vi "LINX - Blink - TCP Interface.vi"() -> ()   [LabVIEW 2011, in "LVH-LINX.lvlib"]
doc: "Blink and LED attached to a digital output channel of a LINX device."
uses:
  vi.lib/LabVIEW Hacker/LINX/LVH-LINX.lvlib
  vi.lib/LabVIEW Hacker/LINX/Private/Device/Type Defs/TCP Config.ctl
  vi.lib/LabVIEW Hacker/LINX/Private/Type Defs/Interface.ctl
  vi.lib/LabVIEW Hacker/LINX/Private/Device/Device.lvlib
panel:
  in  "TCP Configuration":T1
  out "LED Value":bool
  in  "Digital Output Channel":u8=13
  out "Loop Rate (Hz)":u32
  in  "Stop Button":bool
  # "LINX Device Settings"
  # "LED Value"
  # "Circuit Schematic"
  # "Blink (TCP Interface)\n\nThis example demonstrates how to blink an LED on a LINX device connected to \nthe host computer using TCP.\n\nInstructions\n1. Select the IP Address  and Port associated with the LINX Device.\n2. Select the Digital Pin connected to the LED.\n3. Click the Run Arrow."
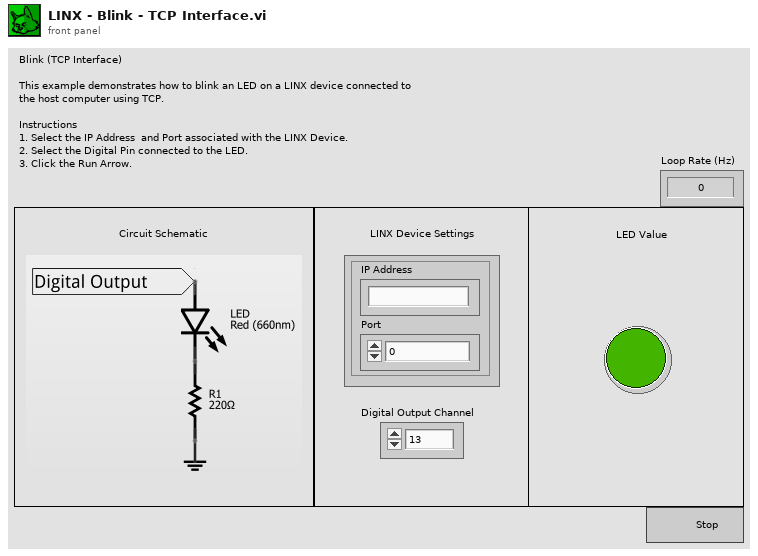
[diagram p1: front panel]
types:
  T1 = typedef "LVH-LINX.lvlib/Device.lvlib/TCP Config.ctl" = cluster{"IP Address":string, "Port":u16}
  T2 = typedef "LVH-LINX.lvlib/Interface.ctl" = enum16{"Serial", "TCP"}
  T3 = typedef "LVH-LINX.lvlib/LINX Ref.ctl" = cluster{"Platform":T4, "Interface":T2, "LINX Device Config":T5}
  T4 = typedef "LVH-LINX.lvlib/Platform.ctl" = enum16{"LINX", "myRIO"}
  T5 = typedef "LVH-LINX.lvlib/Device.lvlib/LINX Device Config.ctl" = cluster{"Interface":T2, "COM Port":refnum<visa-resource-name>, "TCP Configuration":T1, "Device Family":T6, "Device ID":u8, "Device Name":string, "TCP Ref":refnum<k5>}
  T6 = typedef "LVH-LINX.lvlib/Device Family.ctl" = enum8{"National Instruments", "Digilent", "Arduino"}
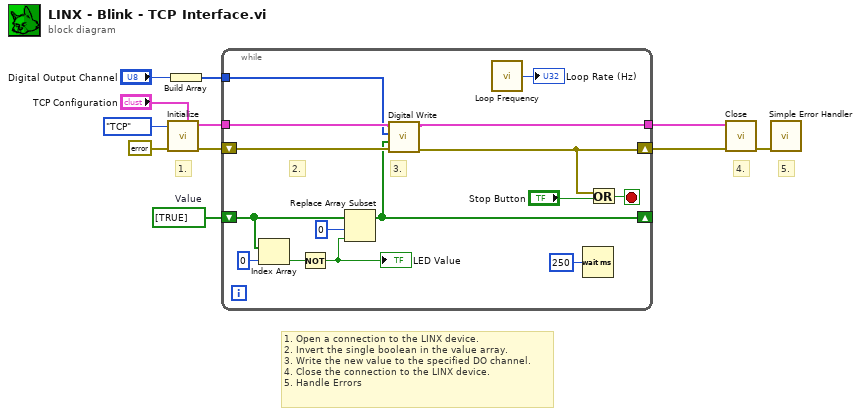
[diagram p0: block diagram]
diagram:
  w4 = bool[] [TRUE]  # Value
  # "1. Open a connection to the LINX device.\n2. Invert the single boolean in the value array.\n3. Write the new value to the specified DO channel.\n4. Close the connection to the LINX device.\n5. Handle Errors"
  # "5."
  # "4."
  # "1."
  n1 = call "Initialize.vi"("TCP Configuration"="TCP Configuration", "Error In"=errorcluster {"status"=FALSE, "code"=0, "source"=""}, "Interface"=Interface."TCP") -> ("Error Out"=w10:errorcluster, "LINX Ref"=w11:T3)  [unwired: 6 in, 1 out]
  n2 = Build Array("Digital Output Channel") -> (w5:u8[])
  n3 = while {
    tunnel: w11 -> [w25]
    tunnel: [w24] -> w9
    shift-right: [w22] -> w8
    shift-left: w10 -> [w23]
    tunnel: w5 -> [w21]
    shift-right: [w16] -> _
    shift-left: w4 -> [w20]
    stop <- w26 stop-if-true
    # "2."
    # "3."
    n4 = Index Array(array=w20, index=0) -> (element=w18:bool)
    n5 = Not(x=w18) -> (.not. x?=w14:bool)
    "LED Value" <- w14
    n6 = Replace Array Subset(array=w20, new element=w14, index=0) -> (w16:bool[])
    n7 = call "Digital Write.vi"("Error In"=w23, "Values"=w16, "DO Channels"=w21, "LINX Resource"=w25) -> ("Error Out"=w22:errorcluster, "LINX Resource"=w24:T3)  [unwired: 6 in]
    n8 = call "Loop Frequency.vi"() -> ("Loop Rate (Hz)"=→"Loop Rate (Hz)":u32)
    n9 = Wait (ms)(milliseconds to wait=u32 250) -> ()  [unwired: 1 out]
    n10 = Or(x=w22, y="Stop Button") -> (x .or. y?=w26:bool)
  }
  n11 = call "Close.vi"("Error In"=w8, "LINX Resource"=w9) -> ("Error Out"=w7:errorcluster)  [unwired: 8 in, 1 out]
  n12 = call <vilib>:"Simple Error Handler.vi"("error in (no error)"=w7) -> ()  [unwired: 4 in, 5 out]
